vi "create glyph manager.vi"(8 "error in":errorcluster, 11 "tree ref (for default symbols)":refnum<vi>) -> (0 "error out":errorcluster, 3 "glyph manager":T1)   [LabVIEW 2025, in "CEF.lvlib"]
doc: "Copyright 2017 National Instruments Corporation\n\nLicensed under the Apache License, Version 2.0 (the \"License\"); you may not use this file except in compliance with the License. You may obtain a copy of the License at http://www.apache.org/licenses/LICENSE-2.0\nUnless required by applicable law or agreed to in writing, software distributed under the License is distributed on an \"AS IS\" BASIS, WITHOUT WARRANTIES OR CONDITIONS OF ANY KIND, either express or implied. See the License for the specific language governing permissions and limitations under the License."
uses:
  CEF.lvlib
  glyph manager.ctl
  <vilib>/picture/picture.llb/imagedata.ctl
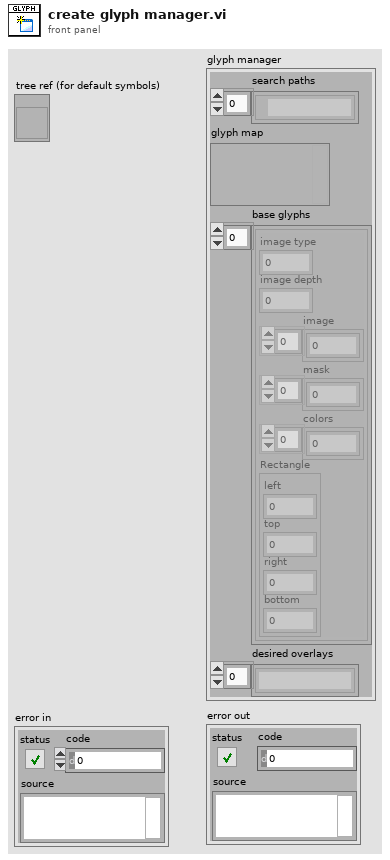
[diagram p1: front panel]
types:
  T1 = typedef "CEF.lvlib/glyph manager.ctl" = cluster{"search paths":path[], "glyph map":variant, "base glyphs":T2[], "desired overlays":string[]}
  T2 = typedef "imagedata.ctl" = cluster{"image type":i32, "image depth":i32, "image":u8[], "mask":u8[], "colors":u32[], "Rectangle":cluster{"left":i16, "top":i16, "right":i16, "bottom":i16}}
  T3 = cluster{"image type":i32, "image depth":i32, "image":u8[], "mask":u8[], "colors":u32[], "Rectangle":cluster{"left":i16, "top":i16, "right":i16, "bottom":i16}}[]
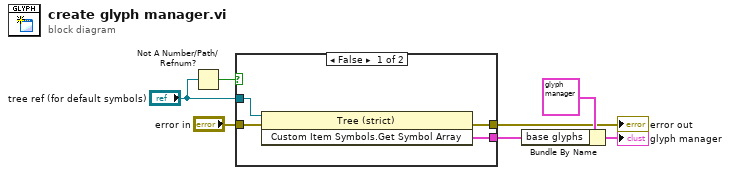
[diagram p0: block diagram]
diagram:
  n1 = Not A Number/Path/Refnum?(number/path/refnum="tree ref (for default symbols)") -> (NaN/Path/Refnum?=w1:bool)
  n2 = case shown="False" w1 {
    tunnel: [w11 _] -> w6
    tunnel: "error in" -> [w10 w12]
    tunnel: [w9 w12] -> w4
    tunnel: "tree ref (for default symbols)" -> [w8 _]
    frame False {
      n3 = invoke class="Tree (strict)" method="Custom Item Symbols.Get Symbol Array"(reference=w8, error in=w10) -> (error out=w9:errorcluster, "Custom Glyphs:Get Glyph Array"=w11:T3)  [unwired: 1 in, 1 out]
    }
    frame True {
    }
  }
  "error out" <- w4
  n4 = Bundle By Name(cluster=T1 {"search paths"=[], "glyph map"=variant, "base glyphs"=[], "desired overlays"=[]} ("glyph manager"), "base glyphs"=w6) -> (→"glyph manager":T1)
